vi "Get Keywords.vi"(8 "error in (no error)":errorcluster, 11 "Timing Functions in":refnum<class "Timing Functions.lvclass">) -> (0 "error out":errorcluster, 2 "Keywords":string[](array[string]), 3 "Timing Functions out":refnum<class "Timing Functions.lvclass">)   [LabVIEW 2016, in "Timing Functions.lvclass"]
uses:
  Timing Functions.lvclass
  functionsbase/functionbase.lvclass
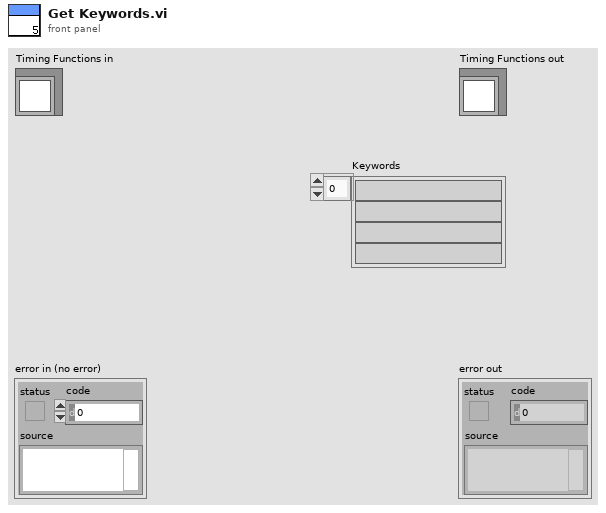
[diagram p1: front panel]
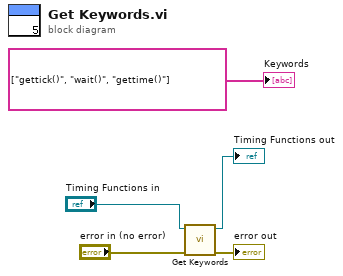
[diagram p0: block diagram]
diagram:
  n1 = call-parent "Get Keywords.vi"("error in (no error)"="error in (no error)", "functionbase in"="Timing Functions in") -> ("error out"=→"error out":errorcluster, "functionbase out"=→"Timing Functions out":refnum<class "Timing Functions.lvclass">)  [unwired: 7 in, 1 out]
  "Keywords" <- string[] ["gettick()", "wait()", "gettime()"] ("Keywords")
